vi "Build Create.vi"(8 "error in (no error)":errorcluster, 9 "tableName":string, 10 "DynamicParameters in":refnum<class "DynamicParameters.lvclass">, 11 "DbConnection in":refnum<class "DbConnection.lvclass">) -> (0 "error out":errorcluster, 1 "LastIdentityQuery":string, 2 "InsertStatement":string, 3 "DbConnection out":refnum<class "DbConnection.lvclass">)   [LabVIEW 2020, in "ORM.lvlib" / "DbConnection.lvclass"]
uses:
  DbConnection.lvclass
  DynamicParameters/DynamicParameters.lvclass
  DynamicParameters/DynamicParameters.lvclass/DynamicParameters.ctl
  DbConnection.lvclass/DbConnection.ctl
  DynamicParameters/Read ParameterNames.vi
  DynamicParameters/Read FieldNames.vi
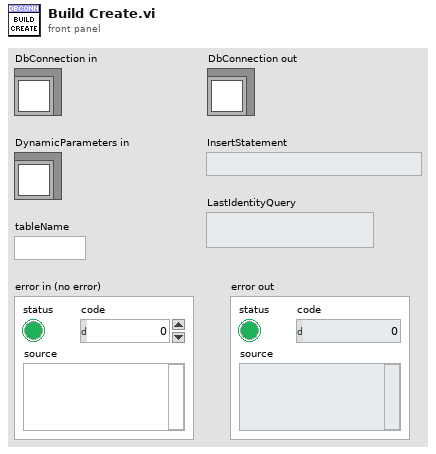
[diagram p1: front panel]
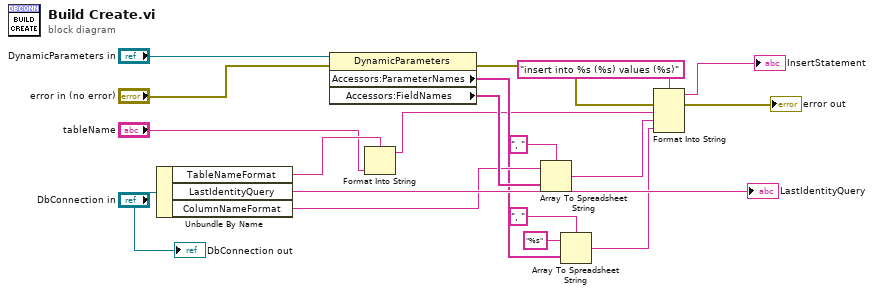
[diagram p0: block diagram]
diagram:
  n1 = Unbundle By Name("DbConnection in") -> ("TableNameFormat"=w3:string, "LastIdentityQuery"=→"LastIdentityQuery":string, "ColumnNameFormat"=w16:string)
  n2 = property class="DynamicParameters"(reference="DynamicParameters in", error in="error in (no error)") -> (error out=w13:errorcluster, "Accessors:ParameterNames"=w7:string[], "Accessors:FieldNames"=w19:string[])  [unwired: 1 out]
  n3 = Format Into String(format string=w3, "tableName") -> (resulting string=w1:string)  [unwired: 2 in, 1 out]
  n4 = Array To Spreadsheet String(delimiter (Tab)=", ", array=w19, 3:w16) -> (spreadsheet string=w11:string)
  n5 = Array To Spreadsheet String(delimiter (Tab)=", ", array=w7, 3:"%s" ("format string")) -> (spreadsheet string=w12:string)
  n6 = Format Into String(format string="insert into %s (%s) values (%s)", error in=w13, w1, w11, w12) -> (resulting string=→"InsertStatement":string, error out=→"error out":errorcluster)  [unwired: 1 in]
  "DbConnection out" <- "DbConnection in"
